vi "ULx Read (Digital Wfm 1Chan NSamp).vi"(0 "task in":refnum<k24>, 7 "number of samples per channel":i32=-1, 9 "timeout":dbl=10.0 format="%_4g", 11 "error in":errorcluster) -> (4 "task out":refnum<k24>, 6 "data":digitalwaveform(waveform), 15 "error out":errorcluster)   [LabVIEW 2020]
doc: "Reads a digital waveform from a task that contains a single digital input channel."
uses:
  C:/Users/William/Documents/LV 2020 builds/LeaktestDAQ/Source-v33/ULx_LV.dll
  ULx_LV.dll
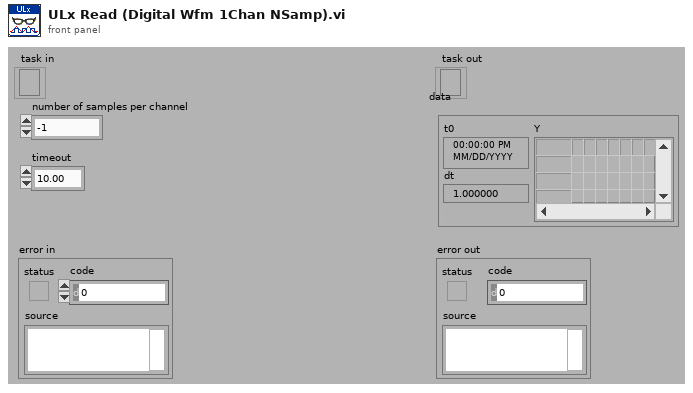
[diagram p1: front panel]
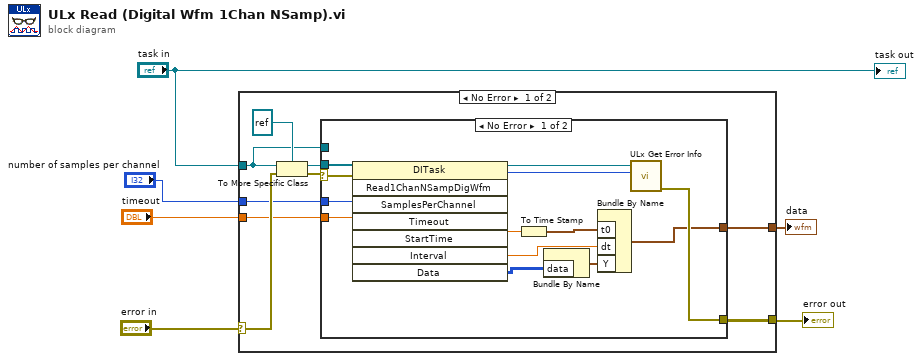
[diagram p0: block diagram]
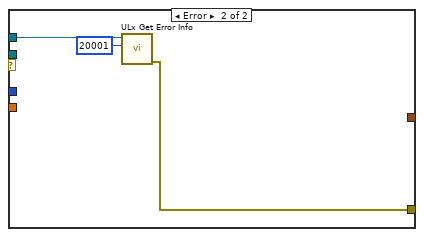
[diagram p2: hidden frame]
diagram:
  n1 = case shown="No Error" "error in" {
    selector: "error in" -> [w15 w32]
    tunnel: "task in" -> [w7 _]
    tunnel: "timeout" -> [w11 _]
    tunnel: [w10 w32] -> w4
    tunnel: [w9 _] -> w2
    tunnel: "number of samples per channel" -> [w8 _]
    frame No Error {
      n2 = To More Specific Class(target class=refnum<k24> refnum, reference=w7, error in=w15) -> (specific class reference=w12:refnum<k24>, error out=w13:errorcluster)
      n3 = case shown="No Error" w13 {
        selector: w13 -> [w27 _]
        tunnel: w12 -> [w28 _]
        tunnel: w11 -> [w18 _]
        tunnel: [w25 w29] -> w10
        tunnel: [w22 _] -> w9
        tunnel: w8 -> [w17 _]
        tunnel: w7 -> [_ w31]
        frame No Error {
          n4 = invoke class="DITask" method="Read1ChanNSampDigWfm"(reference=w28, error in=w27, "SamplesPerChannel"=w17, "Timeout"=w18) -> (reference out=w26:refnum<k24>, "Read1ChanNSampDigWfm"=w16:i32, "StartTime"=w19:dbl, "Interval"=w20:dbl, "Data"=w21:u8[][])  [unwired: 4 in, 3 out]
          n5 = To Time Stamp(1:w19) -> (0:w24:timestamp)
          n6 = Bundle By Name("data"=w21) -> (w23:digitaldata)  [unwired: 1 in]
          n7 = Bundle By Name("t0"=w24, "dt"=w20, "Y"=w23) -> (w22:digitalwaveform)  [unwired: 1 in]
          n8 = call "ULx Get Error Info.vi"("ErrorCode"=w16, "task in"=w26) -> ("error out"=w25:errorcluster)  [unwired: 9 in]
        }
        frame Error {
          n9 = call "ULx Get Error Info.vi"("ErrorCode"=20001, "task in"=w31) -> ("error out"=w29:errorcluster)  [unwired: 9 in]
        }
      }
    }
    frame Error {
    }
  }
  "error out" <- w4
  "data" <- w2
  "task out" <- "task in"
